vi "WaveBook516E Infinite Acquisition.vi"() -> ()   [LabVIEW 2020]
panel:
  out "Waveform Graph":waveform(sgl)(graph)
  out "DAQ #":i32
  out "ScanRate Out":sgl format="%.2f"
  out "Scan List Length":i32
  out "WaveBook516\nChannel Names Out":string[](array[string])
  in  "StartType":T1(ring)=enum."sttImmediate"
  out "Read\nTime Out":bool
  out "Acquisition\nComplete":bool
  in  "WaveBook\n516E Channels":T2={"WaveBook\n516E Channels"=[0], "WaveBook516E\nChannel Names"=["", "", "", "", "", "", "", ""], "Chan Min V"=[-10.0, -10.0, -10.0, -10.0, -10.0, -10.0, -10.0, -10.0], "Chan Max V"=[10.0, 10.0, 10.0, 10.0, 10.0, 10.0, 10.0, 10.0]}
  in  "StopType":T3(ring)=enum."sptManual"
  out "ReturnedScans":i32
  in  "End Acquisition":bool
  in  "Scans to Acquire":i32=100
  in  "ScanRate":sgl=1000.0 format="%.2f"
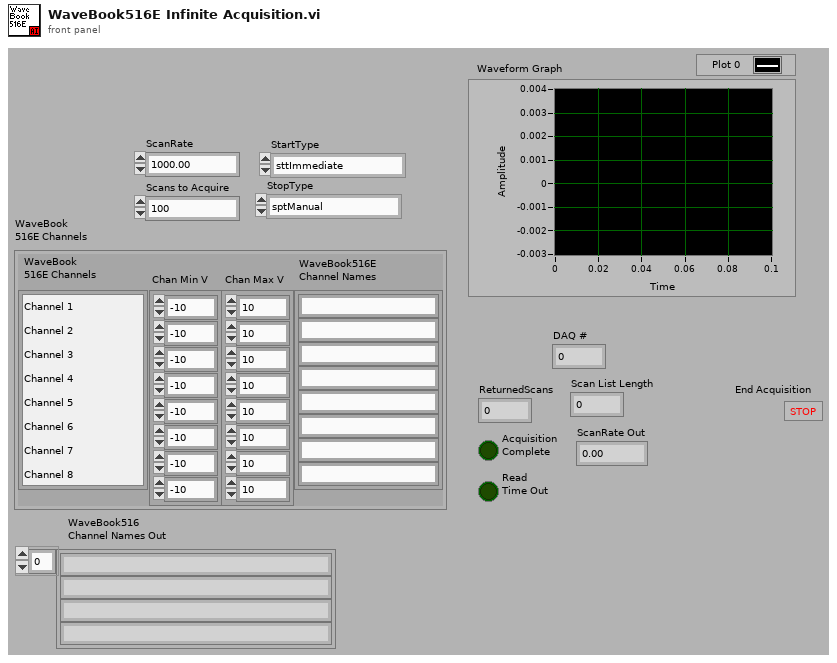
[diagram p1: front panel]
types:
  T1 = enum16{"sttManual", "sttImmediate", "sttMultipleChannel", "sttTTLHigh", "sttTTLLow", "sttTTLRising", "sttTTLFalling", "sttLevelAbove", "sttLevelBelow", "sttEdgeRising", "sttEdgeFalling", "sttLatchedLevelAbove", "sttLatchedLevelBelow", "sttLatchedEdgeRising", "sttLatchedEdgeFalling", "sttWindowInside", "sttWindowOutside", "sttDigitalPatternEQ", "sttDigitalPatternNE", "sttDigitalPatternGT", "sttDigitalPatternLT", "sttHWLevelAbove", "sttHWLevelBelow", "sttHWEdgeRising", "sttHWEdgeFalling"}
  T2 = cluster{"WaveBook\n516E Channels":i32[], "WaveBook516E\nChannel Names":string[], "Chan Min V":dbl[], "Chan Max V":dbl[]}
  T3 = enum16{"sptScanCount", "sptManual", "sptLevelAbove", "sptLevelBelow", "sptEdgeRising", "sptEdgeFalling", "sptWindowInside", "sptWindowOutside", "sptDigitalPatternEQ", "sptDigitalPatternNE", "sptDigitalPatternGT", "sptDigitalPatternLT"}
  T4 = cluster{"Read Timed Out":bool, "Acquisition Complete":bool, "Armed":bool, "Active":bool}
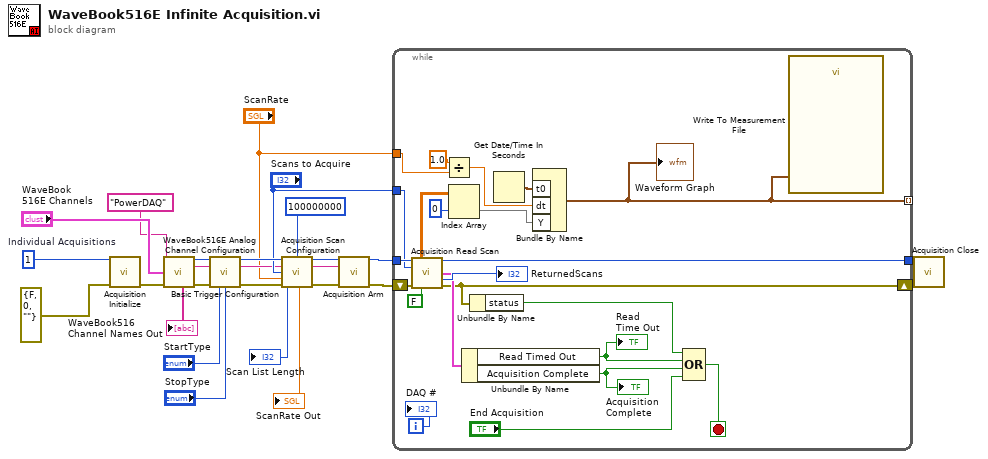
[diagram p0: block diagram]
diagram:
  w14 = 1  # Individual Acquisitions
  n1 = call "Acquisition Initialize.vi"("Individual Acquisitions"=w14, "error in (no error)"=errorcluster {"status"=FALSE, "code"=0, "source"=""}) -> ("error out"=w15:errorcluster)  [unwired: 13 in]
  n2 = call "WaveBook516E Analog Channel Configuration.vi"("DeviceName"="PowerDAQ", "WaveBook516 Channels"="WaveBook\n516E Channels", "error in (no error)"=w15) -> ("Acquisition # OUT"=w26:i16, "DeviceName OUT"=w10:string, "WaveBook516\nChannel Names Out"=→"WaveBook516\nChannel Names Out":string[], "error out"=w25:errorcluster)  [unwired: 8 in, 1 out]
  n3 = call "Basic Trigger Configuration.vi"("Acquisition #"=w26, "DeviceName"=w10, "error in (no error)"=w25, "StartType"="StartType", "StopType"="StopType") -> ("Acquisition #OUT"=w24:i16, "DeviceName OUT"=w8:string, "error out"=w23:errorcluster)  [unwired: 7 in, 1 out]
  n4 = call "Acquisition Scan Configuration.vi"("Acquisition #"=w24, "BufferSize"=100000000, "DeviceName"=w8, "Total Scans to Acquire"="Scans to Acquire", "ScanRate"="ScanRate", "error in (no error)"=w23) -> ("Acquisition #OUT"=w17:i16, "DeviceName OUT"=w7:string, "Scan List Length"=→"Scan List Length":i32, "ScanRate Out"=→"ScanRate Out":sgl, "error out"=w16:errorcluster)  [unwired: 5 in]
  n5 = call "Acquisition Arm.vi"("Acquisition #"=w17, "DeviceName"=w7, "error in (no error)"=w16) -> ("Acquisition #OUT"=w22:i16, "error out"=w21:errorcluster)  [unwired: 9 in, 2 out]
  n6 = while {
    shift-right: [w40] -> w20
    shift-left: w21 -> [w48]
    tunnel: w22 -> [w47]
    tunnel: [w41] -> w19
    tunnel: "Scans to Acquire" -> [w39]
    tunnel: "ScanRate" -> [w31]
    tunnel: [w27] -> _ mode=indexing
    i -> [w28]
    stop <- w45 stop-if-true
    n7 = call "Acquisition Read Scan.vi"("Acquisition #"=w47, "Scans per Iteration"=w39, "error in (no error)"=w48, "Return all\nAvailable Scans"=FALSE ("Return all\nAvailable Scans")) -> ("Acquisition #OUT"=w41:i16, "Returned Data Array"=w35:sgl[][], "Acquisition State"=w43:T4, "Returned Scans"=→"ReturnedScans":i32, "error out"=w40:errorcluster)  [unwired: 6 in, 1 out]
    n8 = Divide(x=sgl 1.0, y=w31) -> (x/y=w29:sgl)
    n9 = Index Array(array=w35, index (col)=0 ("disabled index (col)")) -> (element=w33:sgl[])  [unwired: 1 in]
    n10 = Unbundle By Name(w43) -> ("Read Timed Out"=w37:bool, "Acquisition Complete"=w38:bool)
    "Acquisition\nComplete" <- w38
    "Read\nTime Out" <- w37
    n11 = Unbundle By Name(w40) -> ("status"=w42:bool)
    n12 = Get Date/Time In Seconds() -> (seconds since 1Jan1904=w32:timestamp)
    n13 = Bundle By Name("t0"=w32, "dt"=w29, "Y"=w33) -> (w27:waveform(sgl))  [unwired: 1 in]
    "Waveform Graph" <- w27
    n14 = Compound Arithmetic op=OR(w42, w37, w38, "End Acquisition") -> (w45:bool)
    n15 = call "Write To Measurement File"("Signals"=w27) -> ()  [unwired: 16 in, 3 out]
    "DAQ #" <- w28
  }
  n16 = call "Acquisition Close.vi"("Acquisition #"=w19, "error in (no error)"=w20) -> ()  [unwired: 12 in, 2 out]
